vi "Cleanup_IMU_Interrupt.vi"(6 "error in (no error)":errorcluster, 8 "Event Registration Refnum 2":refnum<event-registration>, 9 "IMU Event":refnum<user-event>) -> (3 "Stop Local Variabl":bool)   [LabVIEW 2014]
uses:
  Interrupt/LV/Interrupt.lvlib
  <userlib>/UCSD Robotics Lab/Robotics-Cape/LV/libroboticscape.lvlib
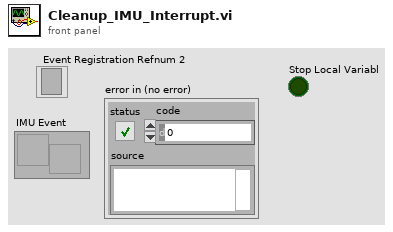
[diagram p1: front panel]
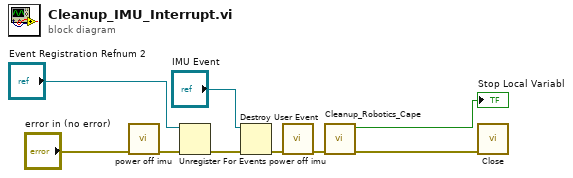
[diagram p0: block diagram]
diagram:
  n1 = call <userlib>:"power off imu.vi"("error in (no error)"="error in (no error)") -> ("error out"=w1:errorcluster)  [unwired: 9 in, 1 out]
  n2 = Unregister For Events(event registration refnum="Event Registration Refnum 2", error in=w1) -> (error out=w8:errorcluster)
  n3 = Destroy User Event(user event="IMU Event", error in=w8) -> (error out=w5:errorcluster)
  n4 = call <userlib>:"power off imu.vi"("error in (no error)"=w5) -> ("error out"=w4:errorcluster)  [unwired: 9 in, 1 out]
  n5 = call "Cleanup_Robotics_Cape.vi"("error in (no error)"=w4) -> ("error out"=w6:errorcluster, "Stop Local Variabl"=→"Stop Local Variabl":bool)  [unwired: 9 in]
  n6 = call "Close.vi"("error in (no error)"=w6) -> ()  [unwired: 9 in, 2 out]
